vi "WriteBaseActor.vi"(7 "ConcreteActor":refnum<class "ConcreteActor.lvclass">, 11 "BaseActor":T1) -> (5 "ConcreteActor":refnum<class "ConcreteActor.lvclass">)   [LabVIEW 2020, in "_Template.lvlib" / "ActorTemplate.lvlib" / "{{Name}}.lvlib" / "ConcreteActor.lvclass"]
uses:
  ConcreteActor.lvclass
  jettl/jettl/Message/Message.lvclass
  ConcreteActor.lvclass/ConcreteActor.ctl
  jettl/jettl/Actor/Actor.lvclass
  jettl/jettl/Lifetime.ctl
  jettl/jettl/jettl.lvlib
  jettl/jettl/MessageSet.ctl
  jettl/jettl/Messages.ctl
  jettl/jettl/Message.ctl
  jettl/jettl/ActorType.ctl
  jettl/jettl/Actor.ctl
  jettl/jettl/ComponentActorMap.ctl
  jettl/jettl/BaseActor.ctl
  jettl/jettl/TellComponentMap.ctl
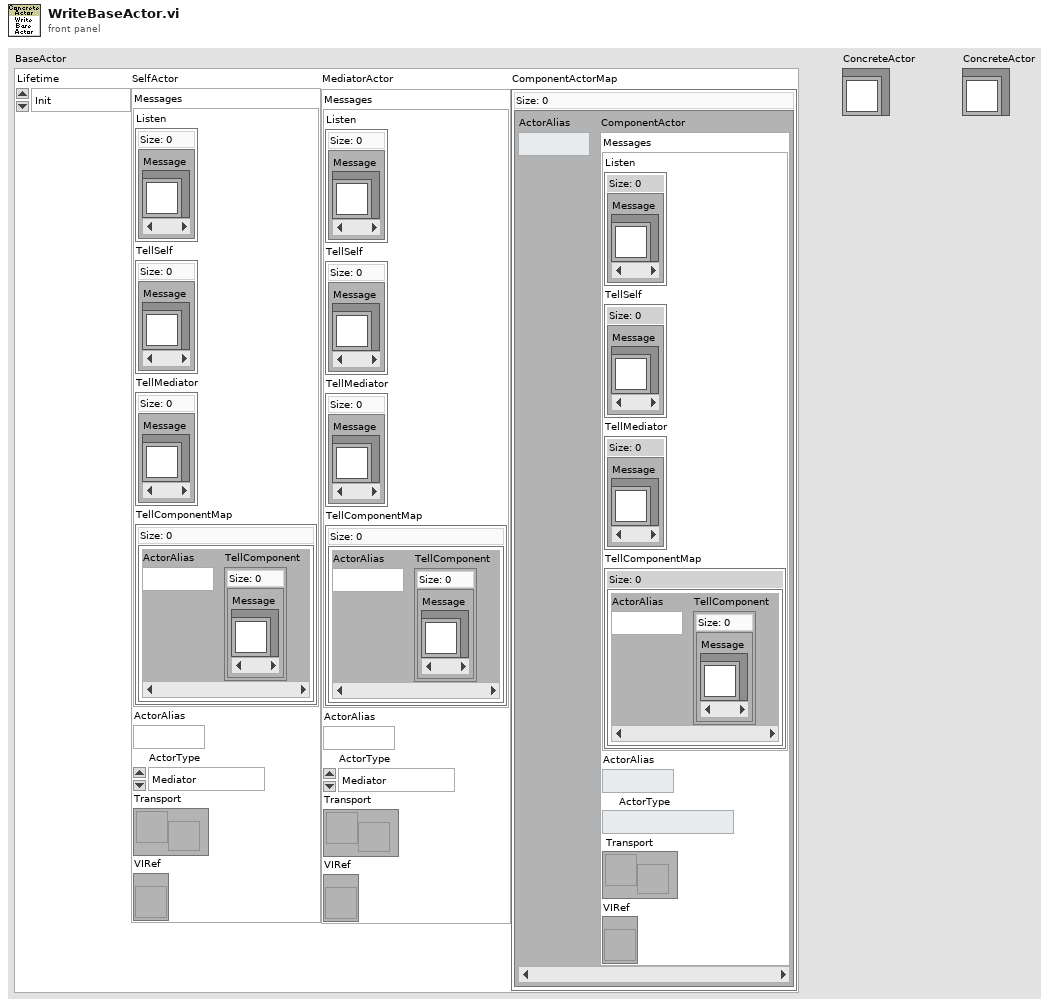
[diagram p1: front panel]
types:
  T1 = typedef "jettl.lvlib/BaseActor.ctl" = cluster{"Lifetime":T2, "SelfActor":T3, "MediatorActor":T3, "ComponentActorMap":T8}
  T2 = typedef "jettl.lvlib/Lifetime.ctl" = enum16{"Init", "Spawn", "Setup", "TeardownBeforeRunning", "Running", "StopCalled", "StoppingWithComponents", "StoppingNoComponents", "TeardownAfterRunning", "Stopped"}
  T3 = typedef "jettl.lvlib/Actor.ctl" = cluster{"Messages":T4, "ActorAlias":string, "ActorType":T7, "Transport":refnum<user-event>, "VIRef":refnum<vi>}
  T4 = typedef "jettl.lvlib/Messages.ctl" = cluster{"Listen":T5, "TellSelf":T5, "TellMediator":T5, "TellComponentMap":T6}
  T5 = typedef "jettl.lvlib/MessageSet.ctl" = set{refnum<class "Message.lvclass">}
  T6 = typedef "jettl.lvlib/TellComponentMap.ctl" = map{string, T5}
  T7 = typedef "jettl.lvlib/ActorType.ctl" = enum16{"Mediator", "Component"}
  T8 = typedef "jettl.lvlib/ComponentActorMap.ctl" = map{string, T3}
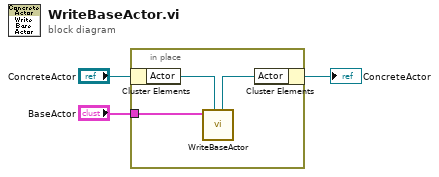
[diagram p0: block diagram]
diagram:
  n1 = in-place {
    in-place-border: "BaseActor" -> [w4]
    n2 = in-place-cluster #1("ConcreteActor") -> ("Actor"=w6:refnum<class "Actor.lvclass">)
    n3 = call-dynamic "WriteBaseActor.vi"("Actor"=w6, "BaseActor"=w4) -> ("Actor"=w5:refnum<class "Actor.lvclass">)  [unwired: 9 in]
    n4 = in-place-cluster #1("Actor"=w5) -> (→"ConcreteActor":refnum<class "ConcreteActor.lvclass">)
  }
